vi "Actor Core.vi"(8 "error in":errorcluster, 11 "Client Actor in":refnum<class "Client Actor.lvclass">) -> (0 "error out":errorcluster, 3 "Actor out":refnum<class "Actor.lvclass">)   [LabVIEW 2019, in "Client Actor.lvlib" / "Client Actor.lvclass"]
doc: "(<B>Filename</B>: Actor Framework.lvlib:Actor.lvclass:Actor Core.vi)\n\nReceives messages to the actor, reacts to them, and initiates any error handling that may shut the actor down.\n\nDescendant classes may override this VI to append parallel tasks for the actor to complete while it handles messages. Overrides use the Call Parent Method node."
uses:
  <vilib>/gpm_packages/@cs/Network-interface/Examples/Client Actor/Client Actor/Client Actor.lvclass
  C:/Program Files/National Instruments/LabVIEW 2019/vi.lib/ActorFramework/Actor/Actor.lvclass
  <vilib>/ActorFramework/Actor/Actor.lvclass
  <vilib>/ActorFramework/Actor/Actor.lvclass/Actor.ctl
  <vilib>/ActorFramework/Message Enqueuer/Message Enqueuer.lvclass/Message Enqueuer.ctl
  <vilib>/gpm_packages/@cs/Network-interface/Source/Network Messenger/Header Data Packet Return/Header Data Packet Return.lvclass/Header Data Packet Return.ctl
  <vilib>/gpm_packages/@cs/Network-interface/Source/Network Messenger/Network Messenger.lvclass/Network Messenger.ctl
  <vilib>/gpm_packages/@cs/Network-interface/Source/Create Ref Message/Create Ref Message.lvclass/Create Ref Message.ctl
  <vilib>/gpm_packages/@cs/Network-interface/Source/Network Messenger/Synchronous Write Callback/Synchronous Write Callback.lvclass/Synchronous Write Callback.ctl
  <vilib>/gpm_packages/@cs/Network-interface/Source/MessagingInterfaces/WriteRequest/WriteRequest.lvclass/WriteRequest.ctl
  <vilib>/gpm_packages/@cs/Network-interface/Source/PersistantConnectionHandler/PersistantConnectionHandler Messages/Execute Write Request Msg/Execute Write Request Msg.lvclass/Execute Write Request Msg.ctl
  <vilib>/gpm_packages/@cs/Network-interface/Source/Network Messenger/Header Data Packet Return/Construct Header Data Packet Return.vi
  <vilib>/gpm_packages/@cs/Network-interface/Source/Create Ref Message/Send Create Reference Message and Wait On Return.vi
  <vilib>/ActorFramework/Message Enqueuer/Init from Existing Queue.vi
  <vilib>/gpm_packages/@cs/Network-interface/Source/PersistantConnectionHandler/PersistantConnectionHandler Messages/Execute Write Request Msg/Send Execute Write Request.vi
  <vilib>/gpm_packages/@cs/Network-interface/Source/MessagingInterfaces/WriteRequest/Pack Write Request.vi
  <vilib>/gpm_packages/@cs/Network-interface/Source/Network Messenger/Synchronous Write Callback/Construct.vi
  <vilib>/gpm_packages/@cs/Network-interface/Source/Network Messenger/Synchronous Write Callback/Wait On Execution.vi
  <vilib>/ActorFramework/Message Enqueuer/Enqueue.vi
  <vilib>/gpm_packages/@cs/Network-interface/Examples/EventMessageRxCallback/EventMessageRxCallback.lvclass
  C:/Program Files/National Instruments/LabVIEW 2019/vi.lib/gpm_packages/@cs/Network-interface/Source/Network Messenger/IPacket Return/IPacket Return.lvclass
  <vilib>/gpm_packages/@cs/Network-interface/Examples/EventConnectionCallback/EventConnectionCallback.lvclass
  C:/Program Files/National Instruments/LabVIEW 2019/vi.lib/gpm_packages/@cs/Network-interface/Source/MessagingInterfaces/IConnectionStateChangeCallback/IConnectionStateChangeCallback.lvclass
  <vilib>/gpm_packages/@cs/Network-interface/Source/Network Messenger/Write Strategy/Write Strategy.lvclass
  C:/Program Files/National Instruments/LabVIEW 2019/vi.lib/gpm_packages/@cs/Network-interface/Source/MessagingInterfaces/IWriteStrategy/IWriteStrategy.lvclass
  <vilib>/gpm_packages/@cs/Network-interface/Source/Network Messenger/ReadStrategy/ReadStrategy.lvclass
  C:/Program Files/National Instruments/LabVIEW 2019/vi.lib/gpm_packages/@cs/Network-interface/Source/MessagingInterfaces/IReadStrategy/IReadStrategy.lvclass
  <vilib>/gpm_packages/@cs/Network-interface/Source/Network Messenger/Header Data Packet Return/Header Data Packet Return.lvclass
  C:/Program Files/National Instruments/LabVIEW 2019/vi.lib/gpm_packages/@cs/Network-interface/Source/MessagingInterfaces/IMessageReturnPolicy/IMessageReturnPolicy.lvclass
  <vilib>/gpm_packages/@cs/Network-interface/Source/TCP Interface/TCP Client/TCP Client.lvclass
  C:/Program Files/National Instruments/LabVIEW 2019/vi.lib/gpm_packages/@cs/Network-interface/Source/IConnectionFactory/IConnectionFactory.lvclass
  <vilib>/gpm_packages/@cs/Network-interface/Source/PersistantConnectionHandler/PersistantConnectionHandler/PersistantConnectionHandler.lvclass
  <vilib>/gpm_packages/@cs/Network-interface/Source/Create Ref Message/Create Ref Message.lvclass
  C:/Program Files/National Instruments/LabVIEW 2019/vi.lib/ActorFramework/Message/Message.lvclass
  <vilib>/gpm_packages/@cs/Network-interface/Source/Network Messenger/Synchronous Write Callback/Synchronous Write Callback.lvclass
  C:/Program Files/National Instruments/LabVIEW 2019/vi.lib/gpm_packages/@cs/Network-interface/Source/MessagingInterfaces/IWriteExecutionCallback/IWriteExecutionCallback.lvclass
  <vilib>/gpm_packages/@cs/Network-interface/Source/Network Messenger/ClusterMessagePacket/ClusterMessagePacket.lvclass
  C:/Program Files/National Instruments/LabVIEW 2019/vi.lib/gpm_packages/@cs/Network-interface/Source/MessagingInterfaces/IPacket/IPacket.lvclass
  <vilib>/gpm_packages/@cs/Network-interface/Source/PersistantConnectionHandler/PersistantConnectionHandler Messages/Execute Write Request Msg/Execute Write Request Msg.lvclass
  <vilib>/ActorFramework/Stop Msg/Stop Msg.lvclass
  <vilib>/gpm_packages/@cs/Network-interface/Source/TCP Interface/TCP Client/Construct TCP Client.vi
  <vilib>/gpm_packages/@cs/Network-interface/Source/PersistantConnectionHandler/PersistantConnectionHandler/Pack Connection Handler.vi
  <vilib>/ActorFramework/Actor/Launch Root Actor.vi
  <vilib>/ActorFramework/Message Priority Queue/Priority Enqueue.vi
  <vilib>/gpm_packages/@cs/Network-interface/Source/Network Messenger/ClusterMessagePacket/Pack.vi
  <vilib>/ActorFramework/Message Enqueuer/Message Enqueuer.lvclass
  <vilib>/gpm_packages/@cs/event-logger/Source/Composed Log/LoggerReference/LoggerReference.lvclass
  <vilib>/gpm_packages/@cs/Network-interface/Source/Network Messenger/Network Messenger.lvclass
  <vilib>/gpm_packages/@cs/Network-interface/Source/MessagingInterfaces/WriteRequest/WriteRequest.lvclass
panel:
  out "Connection":string
  in  "Send":bool
  in  "Message to Send":string
  out "Messages Rx":string
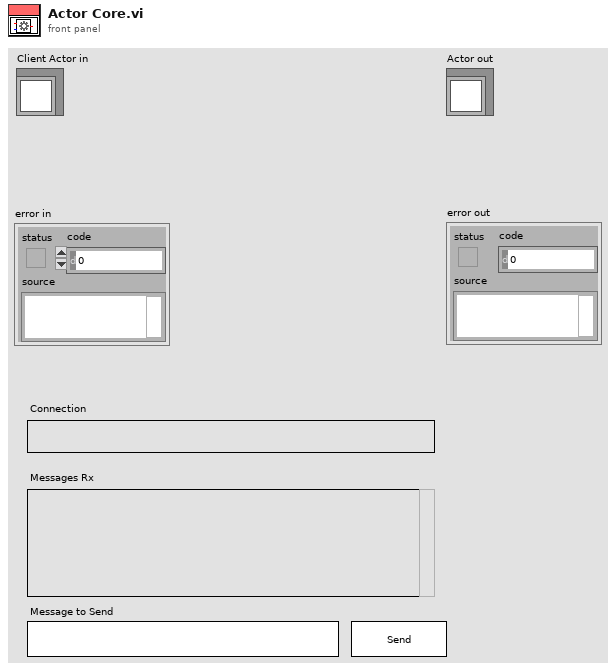
[diagram p1: front panel]
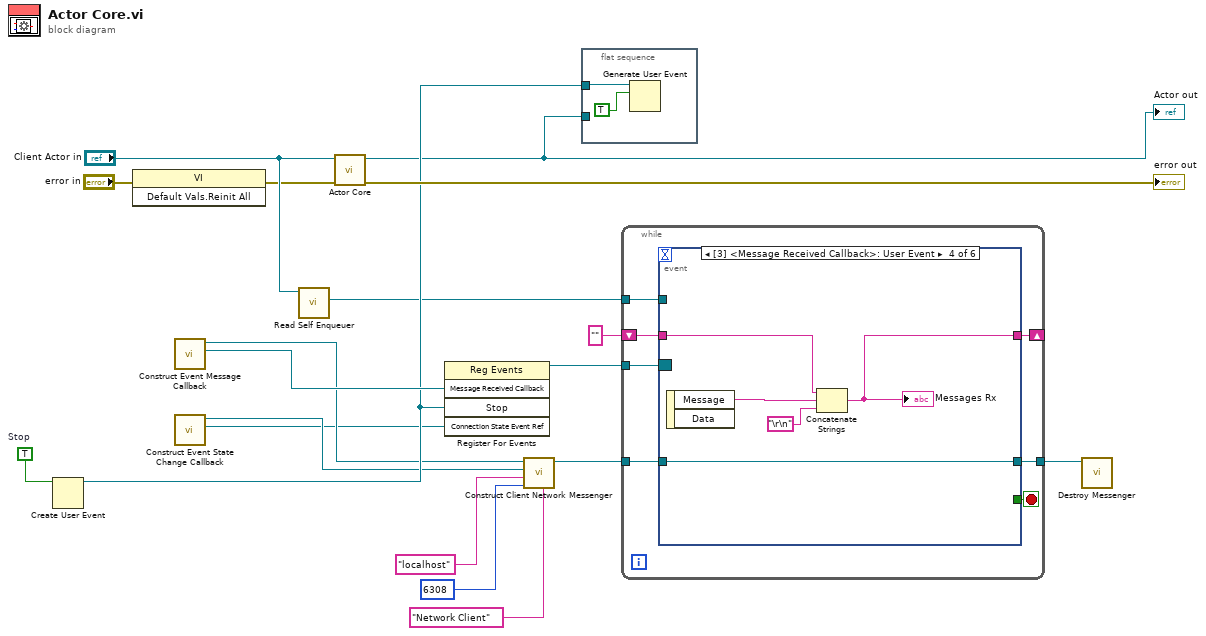
[diagram p0: block diagram]
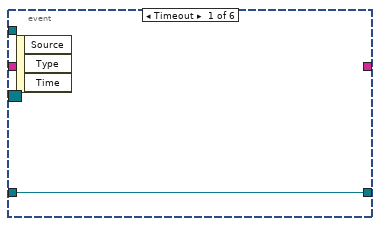
[diagram p2: hidden frame]
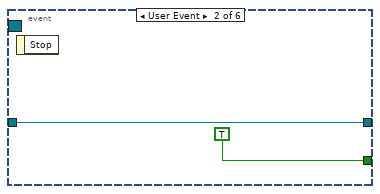
[diagram p3: hidden frame]
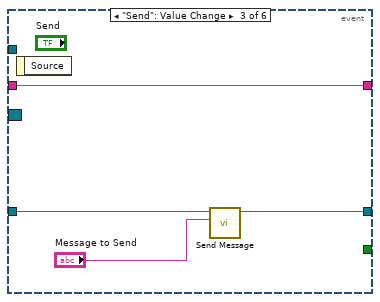
[diagram p4: hidden frame]
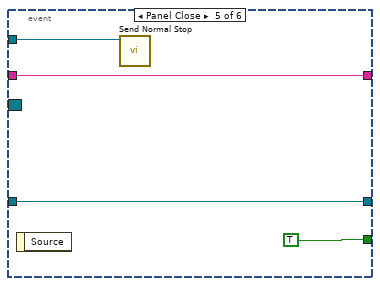
[diagram p5: hidden frame]
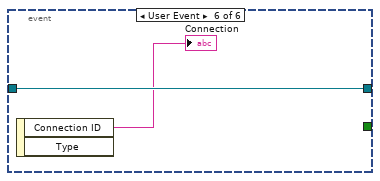
[diagram p6: hidden frame]
diagram:
  w17 = TRUE  # Stop
  n1 = Create User Event(user event datatype=w17) -> (user event=w15:refnum<user-event>)  [unwired: 1 in, 1 out]
  n2 = invoke class="VI" method="Default Vals.Reinit All"(error in="error in") -> (error out=w3:errorcluster)  [unwired: 2 in, 2 out]
  n3 = call <vilib>:"Construct Event Message Callback.vi"() -> ("Message Received Callback"=w18:refnum<user-event>, "EventMessageRxCallback out"=w8:refnum<class "EventMessageRxCallback.lvclass">)  [unwired: 9 in, 1 out]
  n4 = call <vilib>:"Construct Event State Change Callback.vi"() -> ("Connection State Event Ref"=w1:refnum<user-event>, "EventConnectionCallback out"=w2:refnum<class "EventConnectionCallback.lvclass">)  [unwired: 9 in, 1 out]
  n5 = call <vilib>:"Read Self Enqueuer.vi"("Actor"="Client Actor in") -> ("Self Enqueuer"=w12:refnum<class "Message Enqueuer.lvclass">)  [unwired: 10 in]
  n6 = call-parent "Actor Core.vi"("error in"=w3, "Actor in"="Client Actor in") -> ("error out"=→"error out":errorcluster, "Actor out"=w14:refnum<class "Actor.lvclass">)  [unwired: 8 in]
  "Actor out" <- w14
  n7 = register-events(w18, w15, w1) -> (reference out=w16:refnum<event-registration>)  [unwired: 2 in, 1 out]
  n8 = call <vilib>:"Construct Client Network Messenger.vi"("Log Alias"="Network Client", "Remote Port or Service Name"=u16 6308, "Remote IP"="localhost", "Connection State Change Callback"=w2, "Packet Return"=w8) -> ("Network Node"=w7:refnum<data-value>)  [unwired: 5 in, 1 out]
  n9 = flat-sequence {
    tunnel: w15 -> [w21]
    tunnel: w14 -> [_]
    frame #0 {
      n10 = Generate User Event(user event=w21, event data cluster=TRUE) -> ()  [unwired: 2 in, 2 out]
    }
  }
  n11 = while {
    tunnel: w16 -> [w28]
    tunnel: w12 -> [w26]
    tunnel: w7 -> [w25]
    tunnel: [w24] -> w6
    shift-right: [w22] -> _
    shift-left: "" -> [w23]
    stop <- w27 stop-if-true
    n12 = event shown="[3] <Message Received Callback>: User Event" {
      selector: w28 -> [_ _ _ _ _ _]
      dyn-events: _ -> [_ _ _ _ _ _]
      timeout: _ -> [_ _ _ _ _ _]
      tunnel: [_ TRUE _ _ TRUE _] -> w27
      tunnel: w26 -> [_ _ _ _ w43 _]
      tunnel: w25 -> [w29 w30 w35 w40 w42 w46]
      tunnel: [w29 w30 w34 w40 w42 w46] -> w24
      tunnel: w23 -> [_ _ w32 w37 w41 _]
      tunnel: [_ _ w32 w36 w41 _] -> w22
      event Timeout {
        n13 = event-data() -> ()  [unwired: 1 in, 3 out]
      }
      event User Event {
        n14 = event-data() -> ()  [unwired: 1 in, 1 out]
      }
      event "Send": Value Change {
        n15 = event-data() -> ()  [unwired: 1 in, 1 out]
        n16 = call <vilib>:"Send Message.vi"("Message"="Message to Send", "Persistant Network Node In"=w35) -> ("Persistant Network Node Out"=w34:refnum<data-value>)  [unwired: 8 in, 1 out]
      }
      event User Event {
        n17 = event-data() -> ("Message"=w39:string)  [unwired: 1 in, 1 out]
        n18 = Concatenate Strings(w37, w39, "\r\n") -> (w36:string)
        "Messages Rx" <- w36
      }
      event Panel Close {
        n19 = event-data() -> ()  [unwired: 1 in, 1 out]
        n20 = call <vilib>:"Send Normal Stop.vi"("Message Enqueuer"=w43) -> ()  [unwired: 10 in, 1 out]
      }
      event User Event {
        n21 = event-data() -> ("Connection ID"=→"Connection":string)  [unwired: 1 in, 1 out]
      }
    }
  }
  n22 = call <vilib>:"Destroy Messenger.vi"("Network Client Reference In"=w6) -> ()  [unwired: 10 in, 1 out]
